vi "SplitNumber.vi"(11 "x":u32) -> (2 "Lower":u32, 3 "Upper":u32)   [LabVIEW 2009]
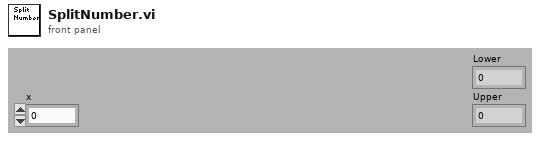
[diagram p1: front panel]
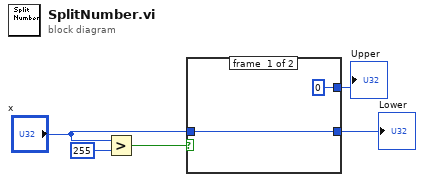
[diagram p0: block diagram]
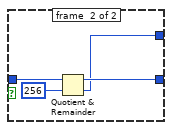
[diagram p2: hidden frame]
diagram:
  n1 = Greater?(x="x", y=u32 255) -> (0:w5:bool)
  n2 = case shown="False" w5 {
    tunnel: "x" -> [w7 w11]
    tunnel: [w7 w10] -> w2
    tunnel: [u32 0 w9] -> w1
    frame #0 {
    }
    frame #1 {
      n3 = Quotient & Remainder(x=w11, y=u32 256) -> (x-y*floor(x/y)=w10:u32, floor(x/y)=w9:u32)
    }
  }
  "Lower" <- w2
  "Upper" <- w1
